vi "New Process (Multiplot).vi"(8 "error in (no error)":errorcluster, 11 "BluePlotHandle in":refnum<class "RocketPlotHandle.lvclass">) -> (0 "error out":errorcluster, 3 "BluePlotHandle out":refnum<class "RocketPlotHandle.lvclass">)   [LabVIEW 2021, in "RocketPlotHandle.lvclass"]
doc: "This will launch a new asynchronous plot instance.\n\n<B>BluePlotHandle in\n</B>This needs to be a user-created object which has dynamic dispatch overrides for satisfying the framework of the package.\n\n<B>Init options</B>\nOptional arguments for affecting the bootup behavior of the plot instance.\nUI Visibile --> Is the UI visible? If no, then the plots are not updated.\nUpdate rate (ms) --> refresh rate of the plots\nvisible sidebar? --> Is the sidebar displaing channel names visible?\ntime to plot (init) --> initial value for the time-to-plot control\ntime to plot (max) --> max allowed entry value for the time-to-plot control\n\n<B>VI ref</B>\nThis output is a reference to the launched plot instance.\nYou are able to insert this into a subpanel, or just open the front panel directly."
uses:
  RocketPlotHandle.lvclass
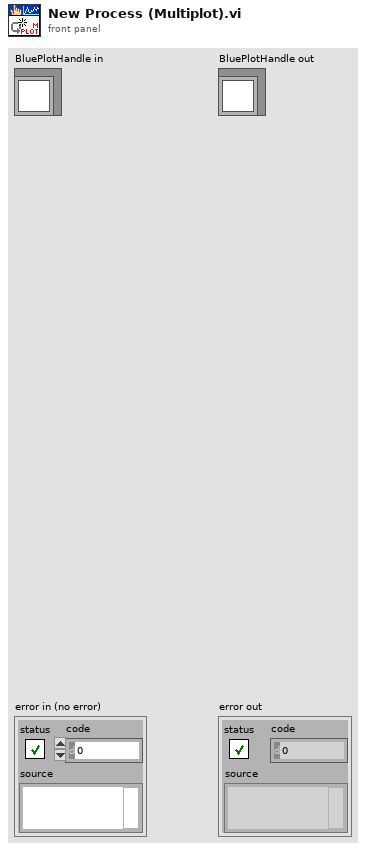
[diagram p1: front panel]
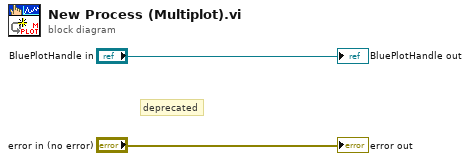
[diagram p0: block diagram]
diagram:
  # "deprecated"
  "error out" <- "error in (no error)"
  "BluePlotHandle out" <- "BluePlotHandle in"
